vi "Pressure Ramp.vi"() -> ()   [LabVIEW 2012]
panel:
  out "Meter":dbl(knob) scale=0.0..10.0
  in  "Slide":dbl(slide) scale=0.0..10.0
  in  "Dial 2":dbl(knob) scale=0.0..100.0
  in  "Dial":dbl(knob) scale=0.0..1.0
  out "Waveform Chart":dynamicdata(graph)
  in  "stop":bool
  out "0-100 PSIG":dbl(knob) caption="PRESSURE GAUGE" scale=0.0..100.0
  out "Pressure (psig)":dbl format="%#_3g"
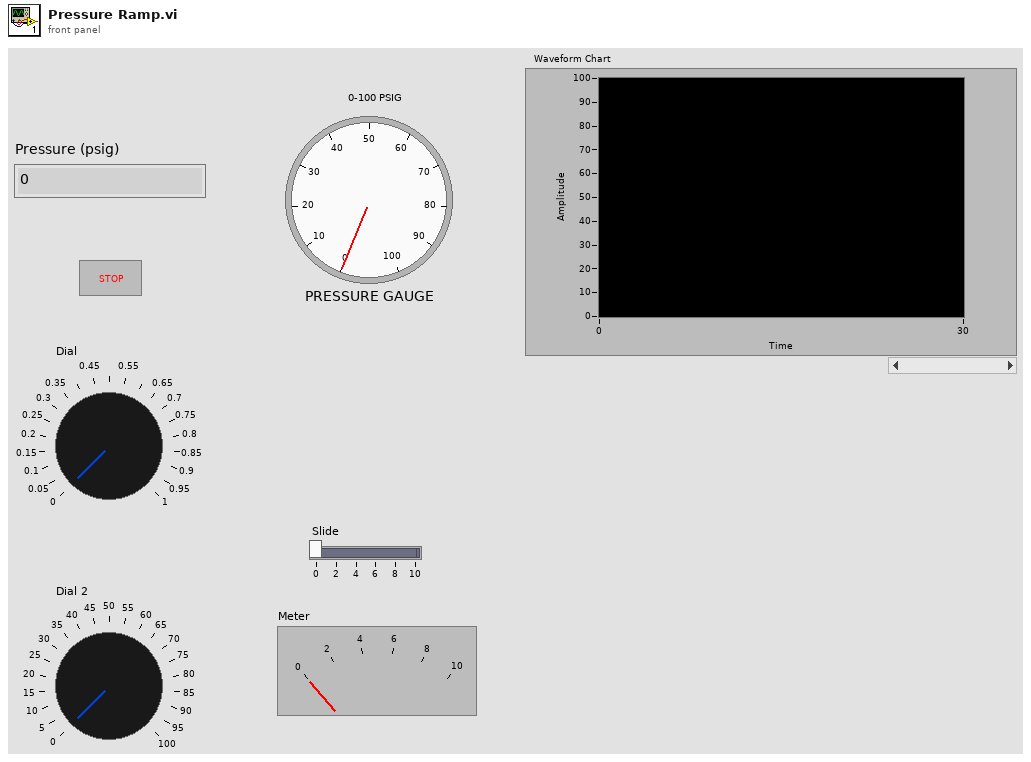
[diagram p1: front panel]
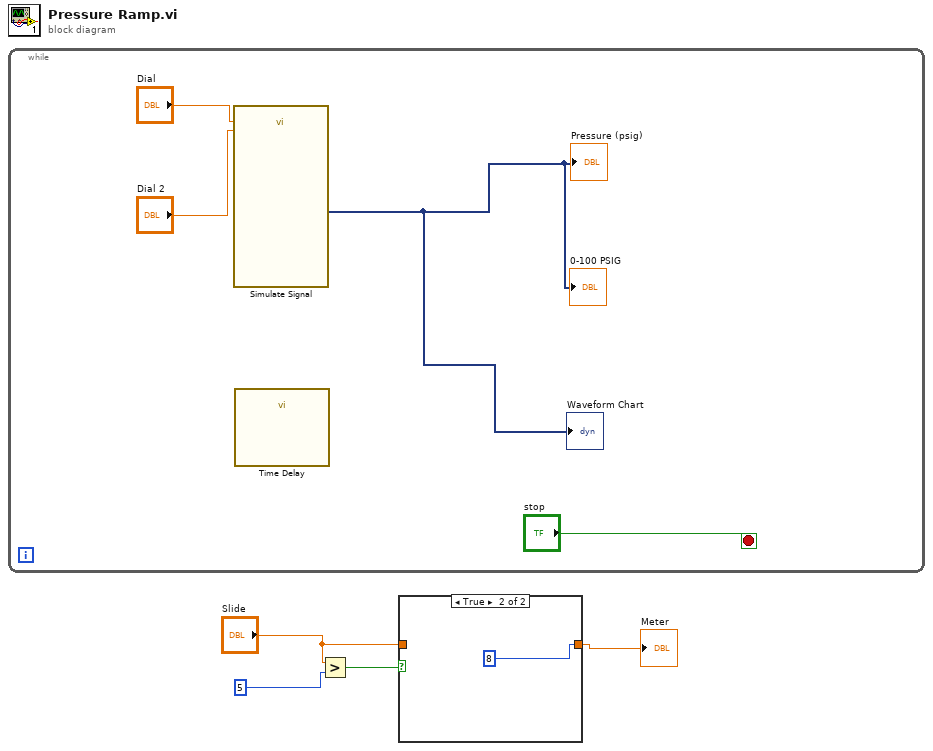
[diagram p0: block diagram]
diagram:
  n1 = while {
    stop <- "stop" stop-if-true
    n2 = call "Simulate Signal"("Frequency"="Dial", "Amplitude"="Dial 2") -> ("Square with Uniform Noise"=→"Pressure (psig)" →"0-100 PSIG" →"Waveform Chart":dynamicdata)  [unwired: 12 in, 1 out]
    n3 = call "Time Delay"() -> ()  [unwired: 11 in, 1 out]
  }
  n4 = Greater?(x="Slide", y=5) -> (0:w3:bool)
  n5 = case shown="True" w3 {
    tunnel: "Slide" -> [w9 _]
    tunnel: [w9 8] -> w1
    frame False {
    }
    frame True {
    }
  }
  "Meter" <- w1
